vi "Initialize.vi"(11 "messengerMbase in":refnum<class "MessengerMBase.lvclass">) -> (3 "messengerMbase out":refnum<class "MessengerMBase.lvclass">)   [LabVIEW 2019, in "MessengerM.lvlib" / "MessengerMBase.lvclass"]
uses:
  MessengerMBase.lvclass
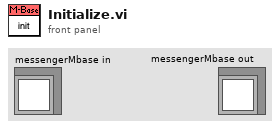
[diagram p1: front panel]
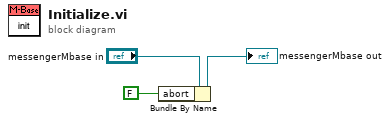
[diagram p0: block diagram]
diagram:
  n1 = Bundle By Name(cluster="messengerMbase in", "abort"=FALSE) -> (→"messengerMbase out":refnum<class "MessengerMBase.lvclass">)
